vi "CANOpen_Main_Cleanup.vi"(0 "interface object":refnum<k20>, 1 "Nodes":T8[](array[typedef]) {"NMT"."Node init static SDO state" items=["start remote node"=1, "enter pre-operational"=128]; "NMT"."Node run state" items=["start remote node"=1, "stop remote node"=2, "enter pre-operational"=128, "reset node"=129, "reset communication"=130]; "Dynamic SDOs"."Sub-Index (0)" format="%.0x"; "Dynamic SDOs"."Object Index" format="%.0x"; "Dynamic SDOs"."Block Data" format="%.0x"; "RPDOs"."PDO Channel" items=["PDO 1", "PDO 2", "PDO 3", "PDO 4"]; "RPDOs"."Parameters"."Bit Offset" max=8 step=1; "RPDOs"."Parameters"."Byte Offset" max=8 step=1; "TPDOs"."PDO Channel" items=["PDO 1", "PDO 2", "PDO 3", "PDO 4"]; "TPDOs"."Parameters"."Bit Offset" max=8 step=1; "TPDOs"."Parameters"."Byte Offset" max=8 step=1; "SDOs"."Sub-Index (0)" format="%.0x"; "SDOs"."Object Index" format="%.0x"; "SDOs"."Block Data" format="%.0x"}, 3 "Enable SYNC":bool, 5 "SYNC object in":refnum<k20>, 9 "xPDO Refs":T5, 10 "SDO queues":T3, 11 "error in (no error)":errorcluster, 12 "Exit":bool, 13 "SDO Asynch":T1 {"HW Dyn Read"."Resp Chan."."Chan Refs" format="%.0x"; "HW Dyn Read"."Req Chan."."Chan Refs" format="%.0x"; "HW Dyn Write"."Resp Chan."."Chan Refs" format="%.0x"; "HW Dyn Write"."Req Chan."."Chan Refs" format="%.0x"; "List SDO"."Resp Chan."."Chan Refs" format="%.0x"; "List SDO"."Req Chan."."Chan Refs" format="%.0x"}, 14 "Security Ref":T4) -> (15 "error out":errorcluster)   [LabVIEW 2021, in "CANOpen Addon Engine.lvlib"]
uses:
  CANOpen Addon Engine.lvlib
  SubVIS/CANOpen_Node Message Settings.ctl
  Shared/CANOpen_PDO Settings.ctl
  Shared/CANOpen_PDO Parameter Settings.ctl
  Shared/CANOpen_PDO Data Type.ctl
  System Explorer/SubVIs/CANopen Byte Order.ctl
  Shared/CANOpen_SDO Settings.ctl
  SubVIS/CANOpen_NMT Settings.ctl
  CanOpen_NMT_Config.ctl
  CanOpen_NMT_Static detect.ctl
  CANOpen_xPDO Refs.ctl
  CanOpen_RPDO Refs.ctl
  CanOpen_TPDO Refs.ctl
  CANOpen_HB_NG_EM Refs.ctl
  CanOpen_SDO queue ref.ctl
  SDO queue.ctl
  SubVIS/CANOpen_VS SDOs Data Refs.ctl
  <vilib>/NI VeriStand/Custom Device API/Data Reference.ctl
  CanOpen_SDO Dynamic queue.ctl
  Shared/CANOpen_SDO queue W data.ctl
  Shared/CANOpen_SDO queue mode.ctl
  Shared/CANOpen_PDO Data Type in queue.ctl
  <vilib>/CANopenLib/CANOPEN.llb/CANopen SYNC Close.vi
  <vilib>/CANopenLib/CANOPEN.llb/CANopen RPDO Close.vi
  <vilib>/CANopenLib/CANOPEN.llb/CANopen TPDO Close.vi
  <vilib>/CANopenLib/CANOPEN.llb/CANopen Create.vi
  <vilib>/CANopenLib/CANOPEN.llb/CANopen SDO Create.vi
  <vilib>/CANopenLib/CANOPEN.llb/CANopen SDO Write.vi
  <vilib>/CANopenLib/CANOPEN.llb/CANopen SDO Write [U16].vi
  <vilib>/CANopenLib/CANOPEN.llb/CANopen SDO Close.vi
  <vilib>/CANopenLib/CANOPEN.llb/CANopen Heartbeat Close.vi
  <vilib>/CANopenLib/CANOPEN.llb/CANopen SDO Write [U8].vi
  <vilib>/CANopenLib/CANOPEN.llb/CANopen Node Guarding Close.vi
  <vilib>/CANopenLib/CANOPEN.llb/CANopen Emergency Close.vi
  <vilib>/CANopenLib/CANOPEN.llb/CANopen Interface Close.vi
  Shared/CANOpen Addon Shared.lvlib
  <vilib>/NI VeriStand/Custom Device API/Custom Device API.lvlib
  System Explorer/CANOpen Addon System Explorer.lvlib
panel:
  # "LSB"
  # "MSB"
  # "LSB"
  # "MSB"
  # "LSB"
  # "MSB"
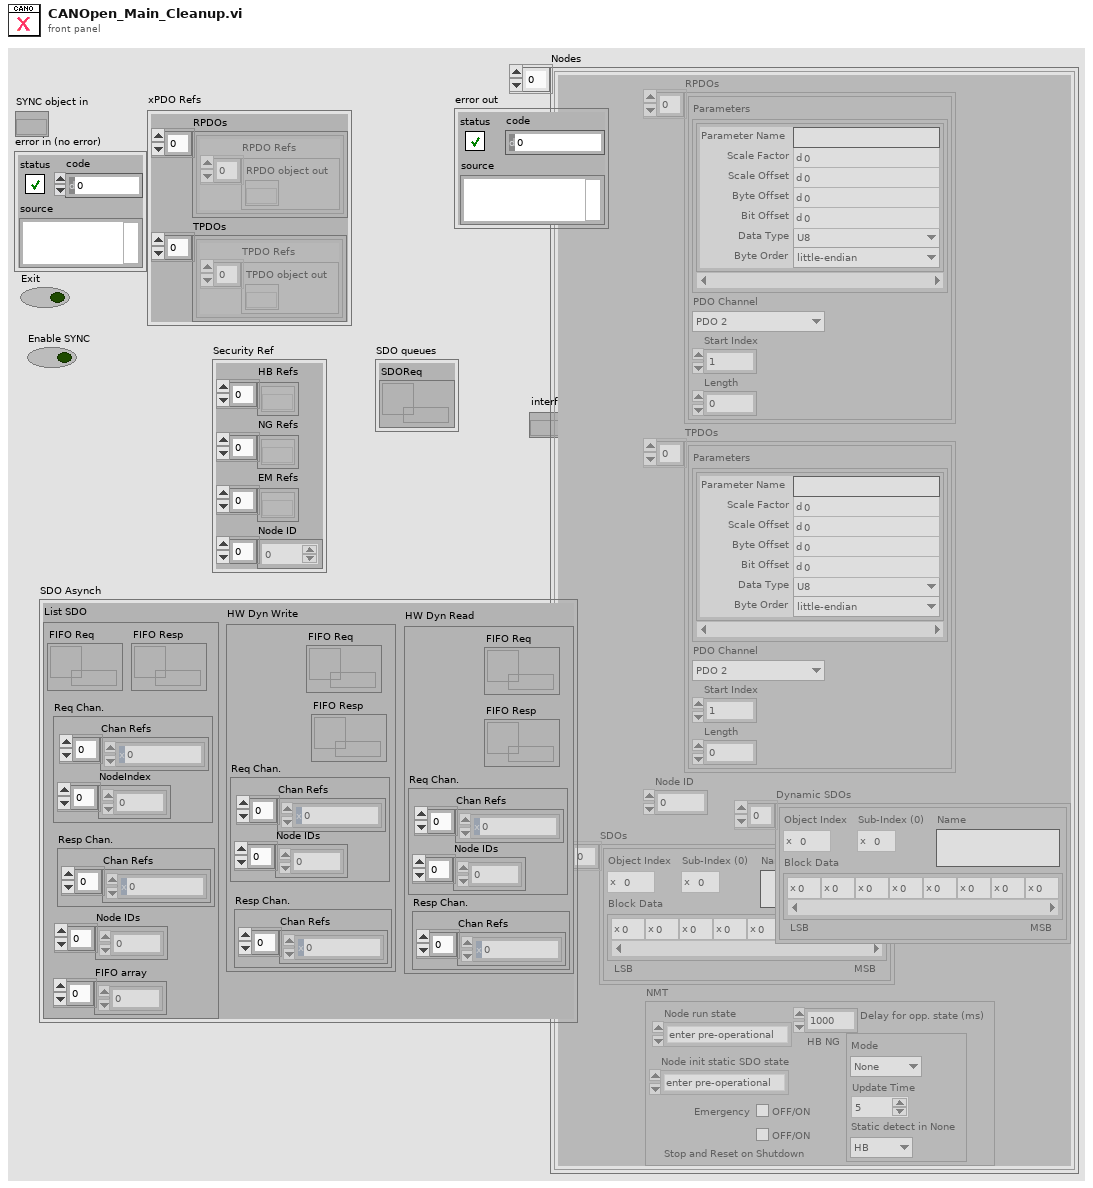
[diagram p1: front panel]
types:
  T1 = typedef "CANOpen Addon Engine.lvlib/CANOpen_VS SDOs Data Refs.ctl" = cluster{"List SDO":cluster{"FIFO Req":refnum<k33>, "Req Chan.":cluster{"Chan Refs":T2[], "NodeIndex":dbl[]}, "FIFO Resp":refnum<k33>, "Resp Chan.":cluster{"Chan Refs":T2[]}, "Node IDs":u8[], "FIFO array":dbl[]}, "HW Dyn Write":cluster{"FIFO Req":refnum<k33>, "FIFO Resp":refnum<k33>, "Req Chan.":cluster{"Chan Refs":T2[], "Node IDs":u8[]}, "Resp Chan.":cluster{"Chan Refs":T2[]}}, "HW Dyn Read":cluster{"FIFO Req":refnum<k33>, "FIFO Resp":refnum<k33>, "Req Chan.":cluster{"Chan Refs":T2[], "Node IDs":u8[]}, "Resp Chan.":cluster{"Chan Refs":T2[]}}}
  T2 = typedef "Custom Device API.lvlib/Data Reference.ctl" = i32
  T3 = typedef "CANOpen Addon Engine.lvlib/CanOpen_SDO queue ref.ctl" = cluster{"SDOReq":refnum<queue>}
  T4 = typedef "CANOpen Addon Engine.lvlib/CANOpen_HB_NG_EM Refs.ctl" = cluster{"HB Refs":refnum<k20>[], "NG Refs":refnum<k20>[], "EM Refs":refnum<k20>[], "Node ID":u8[]}
  T5 = typedef "CANOpen Addon Engine.lvlib/CANOpen_xPDO Refs.ctl" = cluster{"RPDOs":T6[], "TPDOs":T7[]}
  T6 = typedef "CANOpen Addon Engine.lvlib/CanOpen_RPDO Refs.ctl" = cluster{"RPDO Refs":refnum<k20>[]}
  T7 = typedef "CANOpen Addon Engine.lvlib/CanOpen_TPDO Refs.ctl" = cluster{"TPDO Refs":refnum<k20>[]}
  T8 = typedef "CANOpen Addon Engine.lvlib/CANOpen_Node Message Settings.ctl" = cluster{"RPDOs":T9[], "TPDOs":T9[], "Node ID":u8, "SDOs":T13[], "Dynamic SDOs":T13[], "NMT":T14}
  T9 = typedef "CANOpen Addon Shared.lvlib/CANOpen_PDO Settings.ctl" = cluster{"Parameters":T10[], "PDO Channel":u8, "Start Index":u32, "Length":u32}
  T10 = typedef "CANOpen Addon Shared.lvlib/CANOpen_PDO Parameter Settings.ctl" = cluster{"Parameter Name":string, "Scale Factor":dbl, "Scale Offset":dbl, "Byte Offset":u8, "Bit Offset":u8, "Data Type":T11, "Byte Order":T12}
  T11 = typedef "CANOpen Addon Shared.lvlib/CANOpen_PDO Data Type.ctl" = enum16{"U8", "U16", "U32", "I8", "I16", "I32", "Single", "Double", "Boolean"}
  T12 = typedef "CANOpen Addon System Explorer.lvlib/CANopen Byte Order.ctl" = enum16{"big-endian network order", "little-endian"}
  T13 = typedef "CANOpen Addon Shared.lvlib/CANOpen_SDO Settings.ctl" = cluster{"Object Index":u16, "Sub-Index (0)":u8, "Block Data":u8[], "Name":string}
  T14 = typedef "CANOpen Addon Engine.lvlib/CANOpen_NMT Settings.ctl" = cluster{"Node run state":u16, "Emergency":bool, "HB NG":T15, "Delay for opp. state (ms)":dbl, "Node init static SDO state":u16, "Stop and Reset on Shutdown":bool}
  T15 = typedef "CANOpen Addon Engine.lvlib/CanOpen_NMT_Config.ctl" = cluster{"Mode":T16, "Update Time":u16, "Static detect in None":T16}
  T16 = typedef "CANOpen Addon Engine.lvlib/CanOpen_NMT_Static detect.ctl" = enum16{"None", "HB", "NG"}
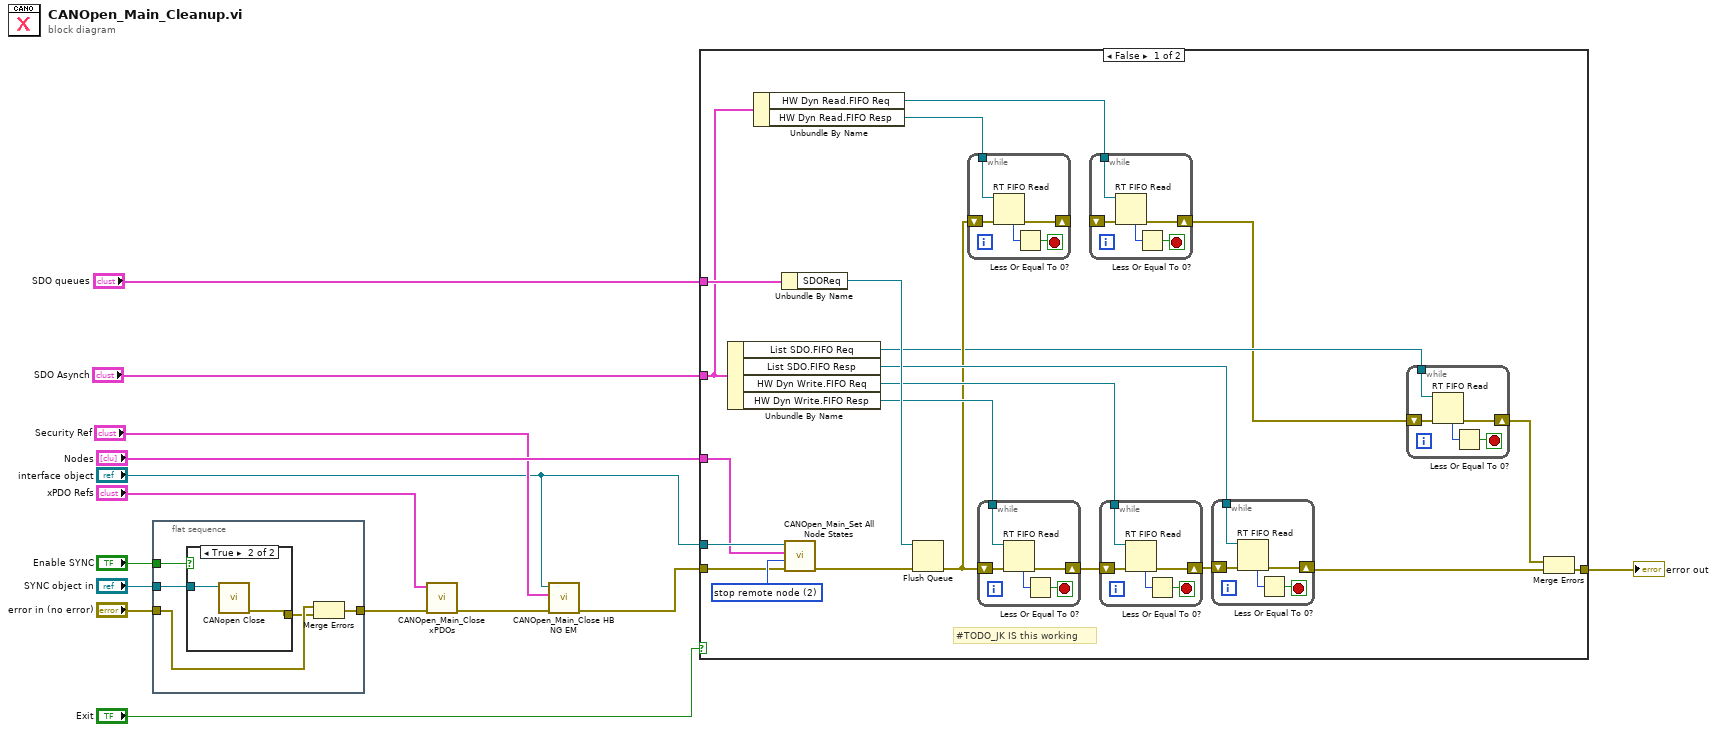
[diagram p0: block diagram]
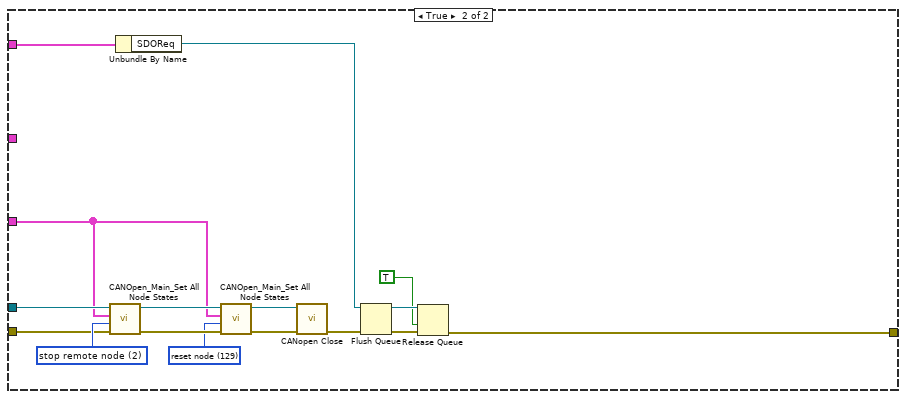
[diagram p3: hidden frame]
diagram:
  n1 = flat-sequence {
    tunnel: [w16] -> w14
    tunnel: "SYNC object in" -> [w19]
    tunnel: "error in (no error)" -> [w18]
    tunnel: "Enable SYNC" -> [w15]
    frame #0 {
      n2 = case shown="True" w15 {
        tunnel: w19 -> [_ w21]
        tunnel: [_ w20] -> w17
        frame False {
        }
        frame True {
          n3 = call-poly <vilib>:"CANopen Close.vi"("SYNC object in"=w21) -> ("error out"=w20:errorcluster)  [unwired: 10 in]
        }
      }
      n4 = Merge Errors(w18, w17) -> (w16:errorcluster)
    }
  }
  n5 = call "CANOpen_Main_Close xPDOs.vi"("error in (no error)"=w14, "xPDO Refs"="xPDO Refs") -> ("error out"=w6:errorcluster)  [unwired: 9 in]
  n6 = call "CANOpen_Main_Close HB NG EM.vi"("error in (no error)"=w6, "Security Ref"="Security Ref", "interface object"="interface object") -> ("error out"=w5:errorcluster)  [unwired: 8 in]
  n7 = case shown="False" "Exit" {
    tunnel: [w32 w73] -> w11
    tunnel: "interface object" -> [w40 w83]
    tunnel: w5 -> [w41 w84]
    tunnel: "Nodes" -> [w39 w82]
    tunnel: "SDO queues" -> [w37 w78]
    tunnel: "SDO Asynch" -> [w28 _]
    frame False {
      w42 = u16 2 items=["start remote node"=1, "stop remote node"=2, "enter pre-operational"=128, "reset node"=129, "reset communication"=130] ("command")
      # "#TODO_JK IS this working"
      n8 = Unbundle By Name(w28) -> ("List SDO.FIFO Req"=w23:refnum<k33>, "List SDO.FIFO Resp"=w29:refnum<k33>, "HW Dyn Write.FIFO Req"=w30:refnum<k33>, "HW Dyn Write.FIFO Resp"=w31:refnum<k33>)
      n9 = Unbundle By Name(w28) -> ("HW Dyn Read.FIFO Req"=w26:refnum<k33>, "HW Dyn Read.FIFO Resp"=w27:refnum<k33>)
      n10 = Unbundle By Name(w37) -> ("SDOReq"=w36:refnum<queue>)
      n11 = call "CANOpen_Main_Set All Node States.vi"("error in (no error)"=w41, "command"=w42, "Nodes"=w39, "interface object"=w40) -> ("error out"=w38:errorcluster)  [unwired: 6 in, 1 out]
      n12 = Flush Queue(queue=w36, error in (no error)=w38) -> (error out=w25:errorcluster)  [unwired: 2 out]
      n13 = while {
        tunnel: w27 -> [w54]
        shift-right: [w53] -> _
        shift-left: w25 -> [w57]
        stop <- w55 stop-if-true
        n14 = RT FIFO Read(0:w54, 3:w57) -> (7:w56:u32, 11:w53:errorcluster)  [unwired: 2 in, 3 out]
        n15 = Less Or Equal To 0?(x=w56) -> (x <= 0?=w55:bool)
      }
      n16 = while {
        tunnel: w31 -> [w69]
        shift-right: [w68] -> w35
        shift-left: w25 -> [w72]
        stop <- w70 stop-if-true
        n17 = RT FIFO Read(0:w69, 3:w72) -> (7:w71:u32, 11:w68:errorcluster)  [unwired: 2 in, 3 out]
        n18 = Less Or Equal To 0?(x=w71) -> (x <= 0?=w70:bool)
      }
      n19 = while {
        tunnel: w26 -> [w49]
        shift-right: [w48] -> w22
        shift-left: _ -> [w52]
        stop <- w50 stop-if-true
        n20 = RT FIFO Read(0:w49, 3:w52) -> (7:w51:u32, 11:w48:errorcluster)  [unwired: 2 in, 3 out]
        n21 = Less Or Equal To 0?(x=w51) -> (x <= 0?=w50:bool)
      }
      n22 = while {
        tunnel: w30 -> [w64]
        shift-right: [w63] -> w34
        shift-left: w35 -> [w67]
        stop <- w65 stop-if-true
        n23 = RT FIFO Read(0:w64, 3:w67) -> (7:w66:u32, 11:w63:errorcluster)  [unwired: 2 in, 3 out]
        n24 = Less Or Equal To 0?(x=w66) -> (x <= 0?=w65:bool)
      }
      n25 = while {
        tunnel: w29 -> [w59]
        shift-right: [w58] -> w33
        shift-left: w34 -> [w62]
        stop <- w60 stop-if-true
        n26 = RT FIFO Read(0:w59, 3:w62) -> (7:w61:u32, 11:w58:errorcluster)  [unwired: 2 in, 3 out]
        n27 = Less Or Equal To 0?(x=w61) -> (x <= 0?=w60:bool)
      }
      n28 = while {
        tunnel: w23 -> [w44]
        shift-right: [w43] -> w24
        shift-left: w22 -> [w47]
        stop <- w45 stop-if-true
        n29 = RT FIFO Read(0:w44, 3:w47) -> (7:w46:u32, 11:w43:errorcluster)  [unwired: 2 in, 3 out]
        n30 = Less Or Equal To 0?(x=w46) -> (x <= 0?=w45:bool)
      }
      n31 = Merge Errors(w24, w33) -> (w32:errorcluster)
    }
    frame True {
      w86 = u16 129 items=["start remote node"=1, "stop remote node"=2, "enter pre-operational"=128, "reset node"=129, "reset communication"=130] ("command")
      w85 = u16 2 items=["start remote node"=1, "stop remote node"=2, "enter pre-operational"=128, "reset node"=129, "reset communication"=130] ("command")
      n32 = call "CANOpen_Main_Set All Node States.vi"("error in (no error)"=w84, "command"=w85, "Nodes"=w82, "interface object"=w83) -> ("error out"=w88:errorcluster, "interface object out"=w87:refnum<k20>)  [unwired: 6 in]
      n33 = Unbundle By Name(w78) -> ("SDOReq"=w75:refnum<queue>)
      n34 = call "CANOpen_Main_Set All Node States.vi"("error in (no error)"=w88, "command"=w86, "Nodes"=w82, "interface object"=w87) -> ("error out"=w81:errorcluster, "interface object out"=w80:refnum<k20>)  [unwired: 6 in]
      n35 = call-poly <vilib>:"CANopen Close.vi"("error in (no error)"=w81, "interface object in"=w80) -> ("error out"=w79:errorcluster)  [unwired: 9 in]
      n36 = Flush Queue(queue=w75, error in (no error)=w79) -> (queue out=w76:refnum<queue>, error out=w77:errorcluster)  [unwired: 1 out]
      n37 = Release Queue(queue=w76, force destroy? (F)=TRUE, error in (no error)=w77) -> (error out=w73:errorcluster)  [unwired: 2 out]
    }
  }
  "error out" <- w11
